vi "6221 AOAI sync.vi"() -> ()   [LabVIEW 2020]
uses:
  <vilib>/DAQmx/write.llb/DAQmx Write (Analog 1D DBL 1Chan NSamp).vi
  <vilib>/DAQmx/read.llb/DAQmx Read (Analog 1D DBL 1Chan NSamp).vi
  <vilib>/DAQmx/create/channels.llb/DAQmx Create Channel (AO-Voltage-Basic).vi
  <vilib>/DAQmx/create/channels.llb/DAQmx Create Channel (AI-Voltage-Basic).vi
  <vilib>/DAQmx/configure/timing.llb/DAQmx Timing (Sample Clock).vi
  <vilib>/DAQmx/configure/trigger.llb/DAQmx Start Trigger (Digital Edge).vi
  <vilib>/DAQmx/miscellaneous.llb/DAQmx Fill In Error Info.vi
  <resource>/objmgr/daqmx.rc
  <vilib>/Analysis/NI_AALBase.lvlib
panel:
  out "Graph":dbl[](graph)
  in  "stop":bool
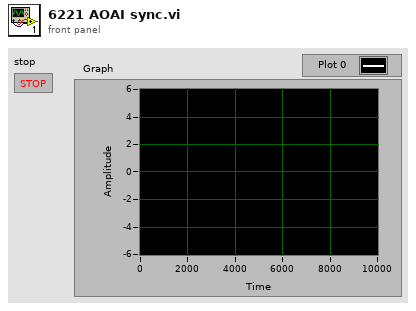
[diagram p1: front panel]
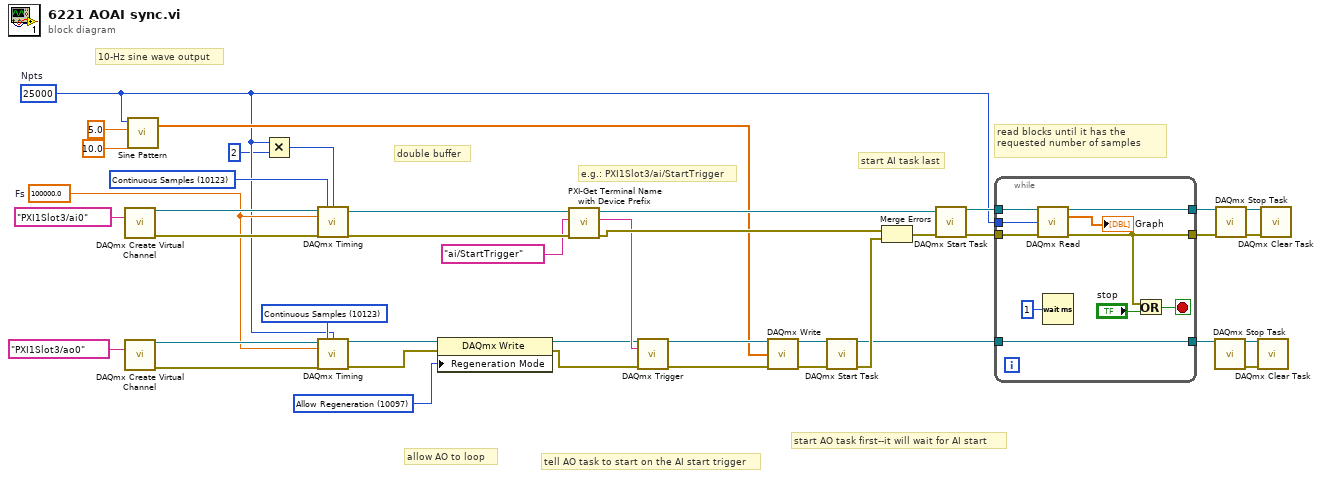
[diagram p0: block diagram]
diagram:
  w12 = 100000.0  # Fs
  w33 = 10123 items=["Finite Samples"=10178, "Continuous Samples"=10123, "Hardware Timed Single Point"=12522] ("sample mode")
  w36 = 10097 items=["Allow Regeneration"=10097, "Do Not Allow Regeneration"=10158] ("RegenMode")
  w3 = 25000  # Npts
  w40 = 10123 items=["Finite Samples"=10178, "Continuous Samples"=10123, "Hardware Timed Single Point"=12522] ("sample mode")
  # "double buffer"
  # "10-Hz sine wave output"
  # "read blocks until it has the requested number of samples"
  # "start AI task last"
  # "start AO task first--it will wait for AI start"
  # "allow AO to loop"
  # "tell AO task to start on the AI start trigger"
  # "e.g.: PXI1Slot3/ai/StartTrigger"
  n1 = call-poly <vilib>:"DAQmx Create Virtual Channel.vi"("physical channels"=tag "PXI1Slot3/ai0") -> ("task out"=w42:refnum<k21>, "error out"=w41:errorcluster)  [unwired: 13 in]
  n2 = call-poly <vilib>:"DAQmx Create Virtual Channel.vi"("physical channels"=tag "PXI1Slot3/ao0") -> ("task out"=w39:refnum<k21>, "error out"=w35:errorcluster)  [unwired: 13 in]
  n3 = call <vilib>:"Sine Pattern.vi"("cycles"=10.0, "amplitude"=5.0, "samples"=w3) -> ("Sinusoidal Pattern"=w4:dbl[])  [unwired: 1 in, 1 out]
  n4 = Multiply(x=w3, y=2) -> (x*y=w1:i32)
  n5 = call-poly <vilib>:"DAQmx Timing.vi"("task/channels in"=w42, "sample mode"=w40, "samples per channel"=w1, "rate"=w12, "error in"=w41) -> ("task out"=w6:refnum<k21>, "error out"=w10:errorcluster)  [unwired: 9 in]
  n6 = call-poly <vilib>:"DAQmx Timing.vi"("task/channels in"=w39, "sample mode"=w33, "samples per channel"=w3, "rate"=w12, "error in"=w35) -> ("task out"=w37:refnum<k21>, "error out"=w38:errorcluster)  [unwired: 9 in]
  n7 = property class="DAQmx Write"(reference=w37, error in=w38, "Regeneration Mode"=w36) -> (reference out=w5:refnum<k21>, error out=w32:errorcluster)
  n8 = call "PXI-Get Terminal Name with Device Prefix.vi"("error in (no error)"=w10, "Local Terminal Name"=tag "ai/StartTrigger" ("source"), "task/channels in"=w6) -> ("error out"=w9:errorcluster, "Terminal Name with Device Prefix"=w7:string, "task out"=w11:refnum<k21>)  [unwired: 6 in]
  n9 = call-poly <vilib>:"DAQmx Trigger.vi"("task/channels in"=w5, "source"=w7, "error in"=w32) -> ("task out"=w18:refnum<k21>, "error out"=w19:errorcluster)  [unwired: 11 in]
  n10 = call-poly <vilib>:"DAQmx Write.vi"("task/channels in"=w18, "data"=w4, "error in"=w19) -> ("task out"=w17:refnum<k21>, "error out"=w16:errorcluster)  [unwired: 10 in, 1 out]
  n11 = call <vilib>:"DAQmx Start Task.vi"("task/channels in"=w17, "error in"=w16) -> ("task out"=w27:refnum<k21>, "error out"=w31:errorcluster)  [unwired: 12 in]
  n12 = Merge Errors(w9, w31) -> (w30:errorcluster)
  n13 = call <vilib>:"DAQmx Start Task.vi"("task/channels in"=w11, "error in"=w30) -> ("task out"=w28:refnum<k21>, "error out"=w29:errorcluster)  [unwired: 12 in]
  n14 = while {
    tunnel: w29 -> [w48]
    tunnel: w28 -> [w49]
    tunnel: w27 -> [w50]
    tunnel: [w47] -> w26
    tunnel: [w43] -> w25
    tunnel: [w50] -> w24
    tunnel: w3 -> [w46]
    stop <- w44 stop-if-true
    n15 = call-poly <vilib>:"DAQmx Read.vi"("task/channels in"=w49, "number of samples per channel"=w46, "error in"=w48) -> ("task out"=w47:refnum<k21>, "data"=→"Graph":dbl[], "error out"=w43:errorcluster)  [unwired: 10 in]
    n16 = Wait (ms)(milliseconds to wait=u32 1) -> ()  [unwired: 1 out]
    n17 = Or(x=w43, y="stop") -> (x .or. y?=w44:bool)
  }
  n18 = call <vilib>:"DAQmx Stop Task.vi"("task/channels in"=w24) -> ("task out"=w21:refnum<k21>, "error out"=w20:errorcluster)  [unwired: 13 in]
  n19 = call <vilib>:"DAQmx Stop Task.vi"("task/channels in"=w26, "error in"=w25) -> ("task out"=w23:refnum<k21>, "error out"=w22:errorcluster)  [unwired: 12 in]
  n20 = call <vilib>:"DAQmx Clear Task.vi"("task in"=w21, "error in"=w20) -> ()  [unwired: 13 in, 1 out]
  n21 = call <vilib>:"DAQmx Clear Task.vi"("task in"=w23, "error in"=w22) -> ()  [unwired: 13 in, 1 out]
